vi "dfd_Inv CH Lowpass S Poles and Zeros.vi"(2 "attenuation (dB)":dbl=60.0 format="%.2f", 3 "low cutoff freq: wl":dbl=0.125 format="%.3f", 4 "order":i32=2) -> (0 "zeros":T1[](array[typedef]), 1 "poles":T1[](array[typedef]))   [LabVIEW 2017, in "NI_DigFilter_Design.lvlib"]
uses:
  <vilib>/addons/Digital Filter Design/NI_DigFilter_Design.lvlib
  <vilib>/addons/Digital Filter Design/_Objects.llb/DFD Pole-Zero.ctl
  <vilib>/addons/Digital Filter Design/NI_DigFilterLicensed.lvlib
panel:
  in  "DFD Zero Pole":T1={"value"=0.0+0.0i, "z attr"={"real"=FALSE, "lp"=FALSE, "uc"=FALSE}, "order"=1}
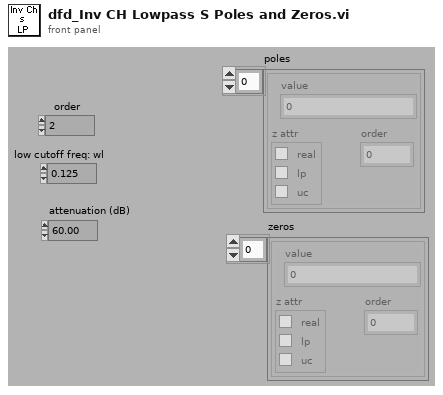
[diagram p1: front panel]
types:
  T1 = typedef "NI_DigFilterLicensed.lvlib/DFD Pole-Zero.ctl" = cluster{"value":cdb, "z attr":cluster{"real":bool, "lp":bool, "uc":bool}, "order":i32}
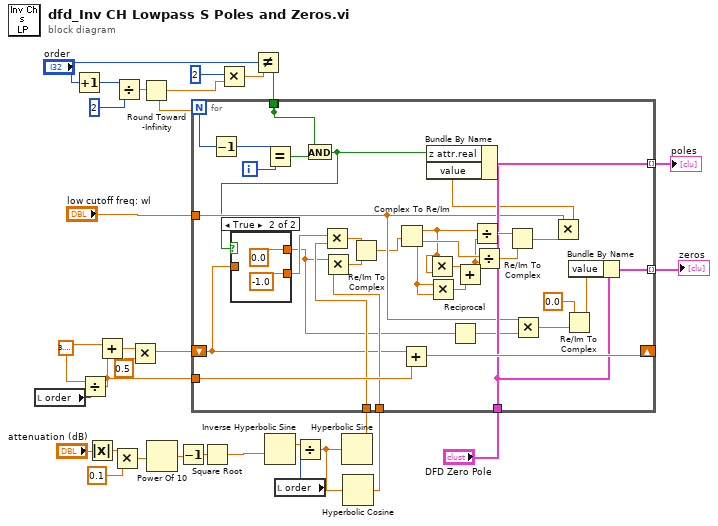
[diagram p0: block diagram]
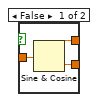
[diagram p2: hidden frame]
diagram:
  w16 = 3.141592653589793
  n1 = local read "order"() -> (w29:i32)
  n2 = Increment(x="order") -> (x+1=w24:i32)
  n3 = Divide(x=w16, y=w29) -> (x/y=w28:dbl)
  n4 = Absolute Value(x="attenuation (dB)") -> (abs(x)=w8:dbl)
  n5 = Add(x=w16, y=w28) -> (x+y=w26:dbl)
  n6 = Multiply(x=w8, y=0.1) -> (x*y=w9:dbl)
  n7 = Divide(x=w24, y=2) -> (x/y=w22:dbl)
  n8 = Multiply(x=w26, y=0.5) -> (x*y=w25:dbl)
  n9 = Round Toward -Infinity(1:w22) -> (0:w17:dbl)
  n10 = Power Of 10(x=w9) -> (10^x=w10:dbl)
  n11 = Decrement(x=w10) -> (x-1=w11:dbl)
  n12 = Square Root(x=w11) -> (sqrt(x)=w1:dbl)
  n13 = Multiply(x=2, y=w17) -> (x*y=w19:dbl)
  n14 = Not Equal?(x="order", y=w19) -> (x != y?=w18:bool)
  n15 = Inverse Hyperbolic Sine(1:w1) -> (0:w12:dbl)
  n16 = local read "order"() -> (w13:i32)
  n17 = Divide(x=w12, y=w13) -> (x/y=w5:dbl)
  n18 = Hyperbolic Sine(1:w5) -> (0:w4:dbl)
  n19 = Hyperbolic Cosine(1:w5) -> (0:w3:dbl)
  n20 = for {
    N: w17 -> [w59]
    shift-right: [w62] -> _
    shift-left: w25 -> [w33]
    tunnel: w28 -> [w63]
    tunnel: "low cutoff freq: wl" -> [w37]
    tunnel: "DFD Zero Pole" -> [w43]
    tunnel: [w56] -> _ mode=indexing
    tunnel: [w57] -> w21 mode=indexing
    tunnel: w18 -> [w56]
    tunnel: w4 -> [w54]
    tunnel: w3 -> [w53]
    tunnel: [w42] -> w2 mode=indexing
    i -> [w61]
    n21 = Decrement(x=w59) -> (x-1=w60:i32)
    n22 = Equal?(x=w60, y=w61) -> (x = y?=w58:bool)
    n23 = And(x=w56, y=w58) -> (x .and. y?=w32:bool)
    n24 = case shown="True" w32 {
      tunnel: w33 -> [w66 _]
      tunnel: [w65 -1.0] -> w55
      tunnel: [w64 0.0] -> w31
      frame False {
        n25 = Sine & Cosine(0:w66) -> (1:w64:dbl, 2:w65:dbl)
      }
      frame True {
      }
    }
    n26 = Multiply(x=w55, y=w54) -> (x*y=w52:dbl)
    n27 = Multiply(x=w31, y=w53) -> (x*y=w51:dbl)
    n28 = Re/Im To Complex(1:w51, 2:w52) -> (0:w36:cdb)
    n29 = Complex To Re/Im(x + iy=w36) -> (x=w46:dbl, y=w50:dbl)
    n30 = Add(x=w33, y=w63) -> (x+y=w62:dbl)
    n31 = Multiply(x=w46, y=w46) -> (x*y=w49:dbl)
    n32 = Multiply(x=w50, y=w50) -> (x*y=w48:dbl)
    n33 = Reciprocal(x=w31) -> (1/x=w39:dbl)
    n34 = Add(x=w49, y=w48) -> (x+y=w47:dbl)
    n35 = Divide(x=w46, y=w47) -> (x/y=w44:dbl)
    n36 = Divide(x=w50, y=w47) -> (x/y=w45:dbl)
    n37 = Re/Im To Complex(1:w45, 2:w44) -> (0:w35:cdb)
    n38 = Multiply(x=w37, y=w39) -> (x*y=w38:dbl)
    n39 = Multiply(x=w37, y=w35) -> (x*y=w34:cdb)
    n40 = Bundle By Name(cluster=w43, "z attr.real"=w32, "value"=w34) -> (w57:T1)
    n41 = Re/Im To Complex(1:w38, 2:0.0) -> (0:w40:cdb)
    n42 = Bundle By Name(cluster=w43, "value"=w40) -> (w42:T1)
  }
  "poles" <- w21
  "zeros" <- w2
